vi "fetch_and_translate_trigger.vi"(8 "error in (no error)":errorcluster, 11 "ImagingModeDL090130Frame in":refnum<class "ImagingModeDL090130Frame.lvclass">) -> (0 "error out":errorcluster, 1 "sender TLC type":T1, 2 "internal trigger":T2, 3 "ImagingModeDL090130Frame out":refnum<class "ImagingModeDL090130Frame.lvclass">)   [LabVIEW 2010, in "ImagingModeDL090130Frame.lvclass"]
uses:
  ImagingModeDL090130Frame.lvclass
  internal_trigger_enum.ctl
  common/enumerations/top-level_component_type_enum.ctl
  GenericImagingMode/GenericImagingMode/trigger_enum.ctl
  common/classes/ErrorController/ErrorController/class_data.vi
  GenericImagingMode/GenericImagingMode/GenericImagingMode.lvclass
  common/classes/ErrorController/ErrorController/ErrorController.lvclass
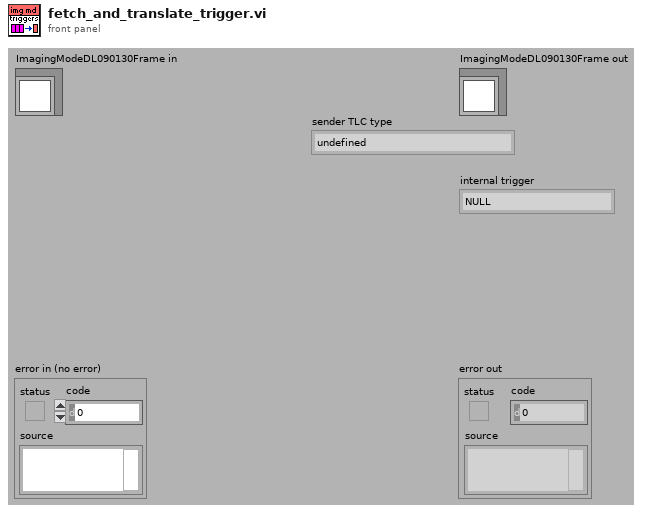
[diagram p1: front panel]
types:
  T1 = typedef "top-level_component_type_enum.ctl" = enum16{"undefined", "ImagingMode", "ScanHead", "DAQ", "ImageAssembler", "Display", "DataCollection", "Analyser", "Stimulator", "ExperimentController", "Instrument", "Stage"}
  T2 = typedef "ImagingModeDL090130Frame.lvclass/internal_trigger_enum.ctl" = enum16{"NULL", "initialise", "terminate", "start", "stop", "proceed", "update", "translate", "start scanning"}
  T3 = typedef "GenericImagingMode.lvclass/trigger_enum.ctl" = enum16{"NULL", "proceed"}
  T4 = typedef "GenericToplevelComponent.lvclass/common_trigger_enum.ctl" = enum16{"NULL", "initialise", "terminate", "fetch command", "fetch data", "attach observer", "register as observer", "detach observer", "acknowledge", "start", "stop", "sweep started", "sweep finished", "experiment started", "experiment stopped"}
  T5 = typedef "trigger_type_enum.ctl" = enum8{"external", "internal", "common"}
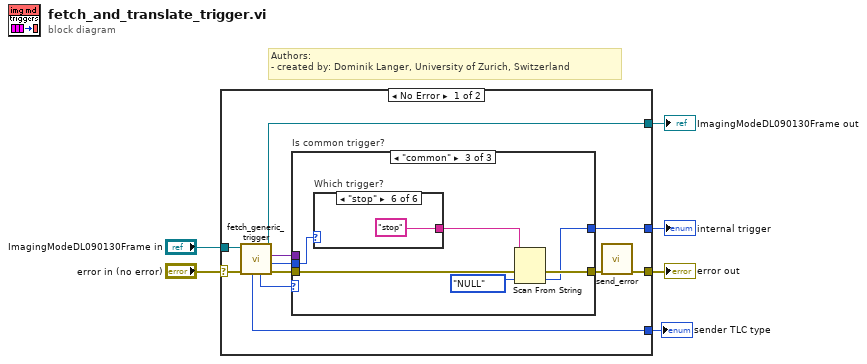
[diagram p0: block diagram]
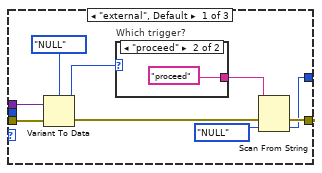
[diagram p2: hidden frame]
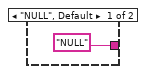
[diagram p3: hidden frame]
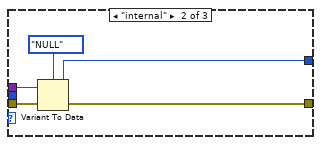
[diagram p4: hidden frame]
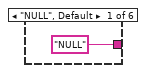
[diagram p5: hidden frame]
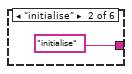
[diagram p6: hidden frame]
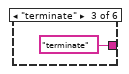
[diagram p7: hidden frame]
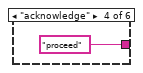
[diagram p8: hidden frame]
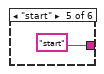
[diagram p9: hidden frame]
diagram:
  # "Authors: \n- created by: Dominik Langer, University of Zurich, Switzerland"
  n1 = case shown="No Error" "error in (no error)" {
    selector: "error in (no error)" -> [w13 w47]
    tunnel: [w17 w47] -> w5
    tunnel: [w14 w46] -> w3
    tunnel: "ImagingModeDL090130Frame in" -> [w15 w46]
    tunnel: [w8 _] -> w2
    tunnel: [w7 _] -> w1
    frame No Error {
      n2 = call-dynamic "fetch_generic_trigger.vi"("error in (no error)"=w13, "GenericToplevelComponent in"=w15) -> ("error out"=w12:errorcluster, "common trigger"=w9:T4, "trigger"=w11:variant, "GenericToplevelComponent out"=w14:refnum<class "ImagingModeDL090130Frame.lvclass">, "trigger type"=w10:T5, "sender TLC type"=w7:T1)  [unwired: 3 in, 1 out]
      n3 = case "Is common trigger?" shown="\"common\"" w10 {
        tunnel: [w19 w30 w36] -> w8
        tunnel: [w21 w32 w38] -> w16
        tunnel: w12 -> [w24 w33 w35]
        tunnel: w11 -> [w23 w31 _]
        tunnel: w9 -> [_ _ w39]
        frame "external", Default {
          n4 = Variant To Data(error in=w24, Variant=w23, type=trigger_enum."NULL" ("message")) -> (error out=w22:errorcluster, data=w26:T3)
          n5 = case "Which trigger?" shown="\"proceed\"" w26 {
            tunnel: ["NULL" "proceed"] -> w18
            frame "NULL", Default {
            }
            frame "proceed" {
            }
          }
          n6 = Scan From String(input string=w18, error in=w22, default 1=internal_trigger_enum."NULL" ("internal trigger")) -> (error out=w21:errorcluster, output 1=w19:T2)  [unwired: 2 in, 2 out]
        }
        frame "internal" {
          n7 = Variant To Data(error in=w33, Variant=w31, type=internal_trigger_enum."NULL" ("internal trigger")) -> (error out=w32:errorcluster, data=w30:T2)
        }
        frame "common" {
          n8 = case "Which trigger?" shown="\"stop\"" w39 {
            tunnel: ["NULL" "initialise" "terminate" "proceed" "start" "stop"] -> w34
            frame "NULL", Default {
            }
            frame "initialise" {
            }
            frame "terminate" {
            }
            frame "acknowledge" {
            }
            frame "start" {
            }
            frame "stop" {
            }
          }
          n9 = Scan From String(input string=w34, error in=w35, default 1=internal_trigger_enum."NULL" ("internal trigger")) -> (error out=w38:errorcluster, output 1=w36:T2)  [unwired: 2 in, 2 out]
        }
      }
      n10 = call "send_error.vi"("error in (no error)"=w16) -> ("error out"=w17:errorcluster)  [unwired: 10 in]
    }
    frame Error {
    }
  }
  "error out" <- w5
  "ImagingModeDL090130Frame out" <- w3
  "internal trigger" <- w2
  "sender TLC type" <- w1
